vi "SQL_param_alarm_select_table.vi"() -> (2 "error out":errorcluster, 3 "表格控件":string[][](table))   [LabVIEW 2014]
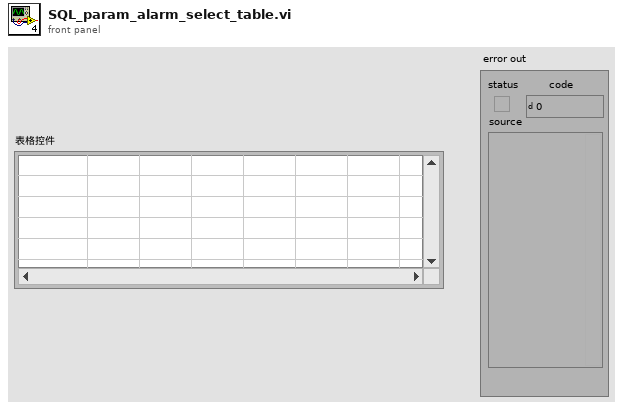
[diagram p1: front panel]
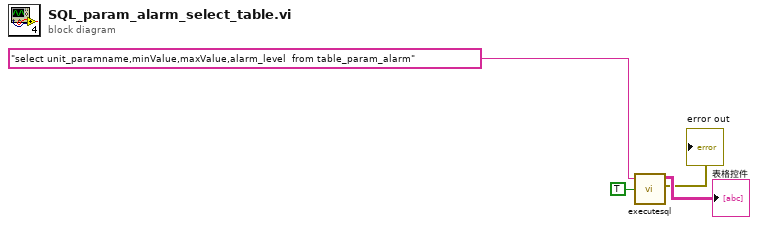
[diagram p0: block diagram]
diagram:
  n1 = call "executesql.vi"("Return Data (T)"=TRUE, "Command Text"="select unit_paramname,minValue,maxValue,alarm_level  from table_param_alarm") -> ("error out"=→"error out":errorcluster, "Data"=→"表格控件":string[][])  [unwired: 5 in]
